vi "CAN Initialize FD.vi"(10 "BitrateFD":string, 11 "Channel":u16) -> (1 "Channel out":u16, 2 "BitrateFD out":string, 3 "function return":u32)   [LabVIEW 2020, in "PCANBasic.lvlib"]
doc: "TPCANStatus __stdcall CAN_InitializeFD(\n TPCANHandle Channel,\n TPCANBitrateFD BitrateFD);"
uses:
  PCANBasic.lvlib
  <userlib>/PCANBasic/PCANBasic.dll
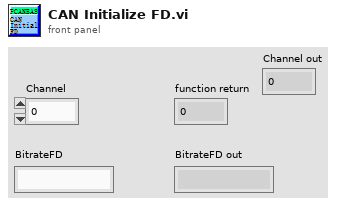
[diagram p1: front panel]
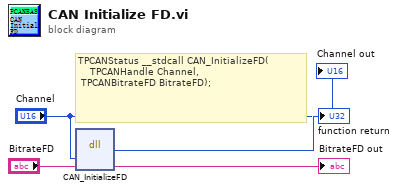
[diagram p0: block diagram]
diagram:
  # "TPCANStatus __stdcall CAN_InitializeFD(\n    TPCANHandle Channel,\n\tTPCANBitrateFD BitrateFD);"
  n1 = dll-call lib="D:/Program Files (x86)/National Instruments/LabVIEW 2020/user.lib/PCANBasic/PCANBasic.*" fn="CAN_InitializeFD"("Channel"="Channel", "BitrateFD"="BitrateFD") -> ("返回类型"=→"function return":u16, "BitrateFD"=→"BitrateFD out":string)  [unwired: 4 in, 2 out]
  "Channel out" <- "Channel"
